vi "Configure Time Domain Transform.vi"(0 "VISA resource name":refnum<visa-resource-name>, 1 "Channel (1)":i32=1, 2 "Transformation Type (0: Band - pass)":u16(ring) items=["Band-pass", "Low-pass"], 3 "Stimulus Type (0: Impulse)":u16(ring) items=["Impulse", "Step"], 5 "Transformation Function State (F: Disable)":bool, 7 "Beta (6)":i32=6, 9 "Impulse Width (0.0)":dbl format="%.2e", 11 "error in (no error)":errorcluster, 12 "Rise Time of Step Signal  (0.0)":dbl format="%.2e") -> (4 "VISA resource name out":refnum<visa-resource-name>, 15 "error out":errorcluster)   [LabVIEW 2018, in "Agilent ENA Series.lvlib"]
doc: "Configures the time domain transformation."
uses:
  Agilent ENA Series.lvlib
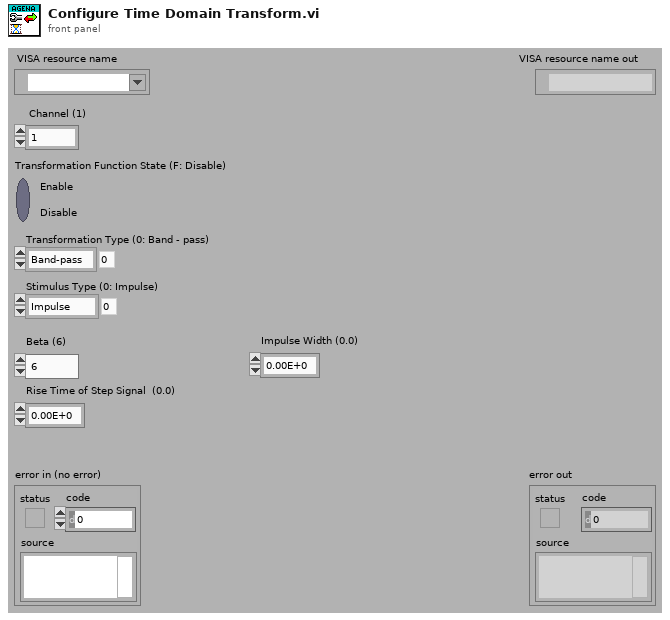
[diagram p1: front panel]
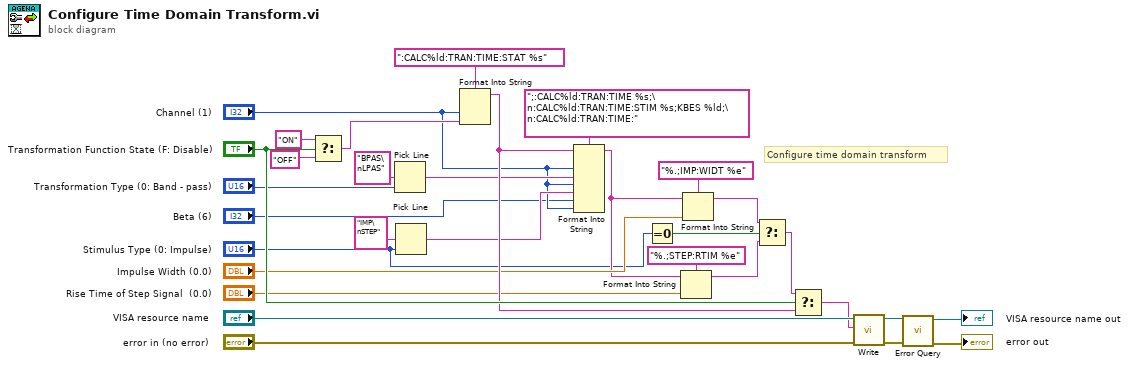
[diagram p0: block diagram]
diagram:
  # "Configure time domain transform"
  n1 = Select(t="ON", s="Transformation Function State (F: Disable)", f="OFF") -> (s? t:f=w26:string)
  n2 = Pick Line(multi-line string="BPAS\nLPAS", line index="Transformation Type (0: Band - pass)") -> (output string=w19:string)  [unwired: 1 in]
  n3 = Pick Line(multi-line string="IMP\nSTEP", line index="Stimulus Type (0: Impulse)") -> (output string=w18:string)  [unwired: 1 in]
  n4 = Format Into String(format string=":CALC%ld:TRAN:TIME:STAT %s", "Channel (1)", w26) -> (resulting string=w23:string)  [unwired: 2 in, 1 out]
  n5 = Format Into String(format string=";:CALC%ld:TRAN:TIME %s;\n:CALC%ld:TRAN:TIME:STIM %s;KBES %ld;\n:CALC%ld:TRAN:TIME:", initial string=w23, "Channel (1)", w19, "Channel (1)", w18, "Beta (6)", "Channel (1)") -> (resulting string=w13:string)  [unwired: 1 in, 1 out]
  n6 = Equal To 0?(x="Stimulus Type (0: Impulse)") -> (x = 0?=w12:bool)
  n7 = Format Into String(format string="%.;STEP:RTIM %e", initial string=w13, "Rise Time of Step Signal  (0.0)") -> (resulting string=w10:string)  [unwired: 1 in, 1 out]
  n8 = Format Into String(format string="%.;IMP:WIDT %e", initial string=w13, "Impulse Width (0.0)") -> (resulting string=w11:string)  [unwired: 1 in, 1 out]
  n9 = Select(t=w11, s=w12, f=w10) -> (s? t:f=w8:string)
  n10 = Select(t=w8, s="Transformation Function State (F: Disable)", f=w23) -> (s? t:f=w7:string)
  n11 = call "Write.vi"("error in (no error)"="error in (no error)", "String ()"=w7, "VISA resource name"="VISA resource name") -> ("error out"=w3:errorcluster, "VISA resource name out"=w4:refnum<visa-resource-name>)  [unwired: 6 in, 1 out]
  n12 = call "Error Query.vi"("error in (no error)"=w3, "VISA resource name"=w4) -> ("error out"=→"error out":errorcluster, "VISA resource name out"=→"VISA resource name out":refnum<visa-resource-name>)  [unwired: 6 in, 2 out]
